vi "Engine Out - Direct Injectors.vi"(7 "Rail Pressure [bar]":sgl, 10 "DI Timings (DBTDC)":T3[](array[typedef]), 11 "DI Quantities (mg/inj)":T2[](array[typedef])) -> (0 "Injector 5":T1, 1 "Injector 6":T1, 2 "Injector 7":T1, 3 "Injector 8":T1, 4 "Injector 4":T1, 6 "Injector 3":T1, 8 "Injector 2":T1, 9 "Injector 1":T1)   [LabVIEW 2015, in "ECS-RT.lvlib"]
uses:
  ECS-RT.lvlib
  Typedefs/Control Outputs/Injection Timing.ctl
  Typedefs/Control Outputs/Injection Quantity.ctl
  Typedefs/Raw Outputs/DI.ctl
  ECS-Shared.lvlib
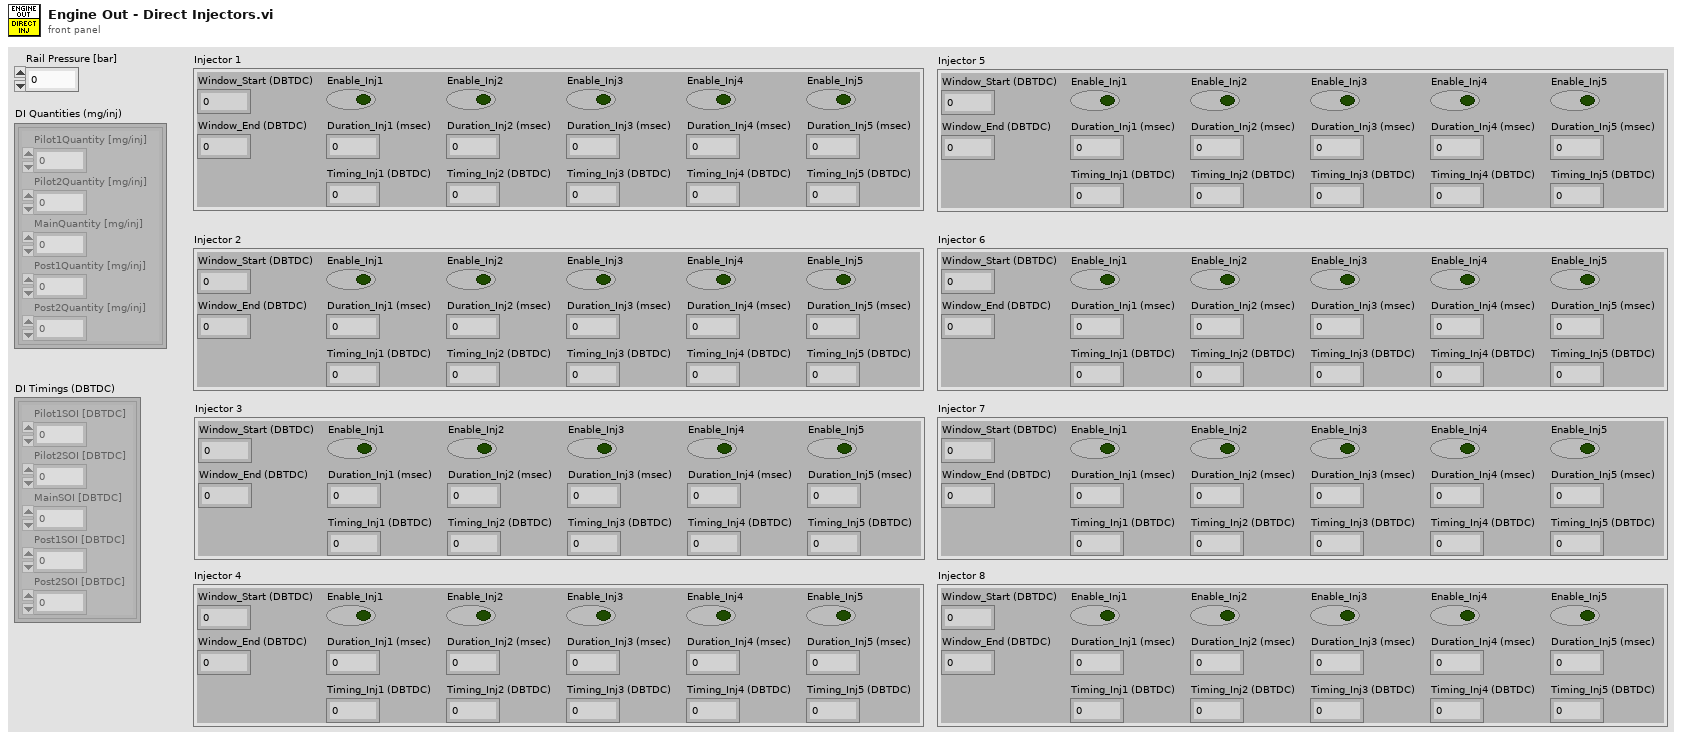
[diagram p1: front panel]
types:
  T1 = typedef "ECS-Shared.lvlib/DI.ctl" = cluster{"Window_Start (DBTDC)":sgl, "Window_End (DBTDC)":sgl, "Enable_Inj1":bool, "Duration_Inj1 (msec)":sgl, "Timing_Inj1 (DBTDC)":sgl, "Enable_Inj2":bool, "Duration_Inj2 (msec)":sgl, "Timing_Inj2 (DBTDC)":sgl, "Enable_Inj3":bool, "Duration_Inj3 (msec)":sgl, "Timing_Inj3 (DBTDC)":sgl, "Enable_Inj4":bool, "Duration_Inj4 (msec)":sgl, "Timing_Inj4 (DBTDC)":sgl, "Enable_Inj5":bool, "Duration_Inj5 (msec)":sgl, "Timing_Inj5 (DBTDC)":sgl}
  T2 = typedef "ECS-Shared.lvlib/Injection Quantity.ctl" = cluster{"Pilot1Quantity [mg/inj]":sgl, "Pilot2Quantity [mg/inj]":sgl, "MainQuantity [mg/inj]":sgl, "Post1Quantity [mg/inj]":sgl, "Post2Quantity [mg/inj]":sgl}
  T3 = typedef "ECS-Shared.lvlib/Injection Timing.ctl" = cluster{"Pilot1SOI [DBTDC]":sgl, "Pilot2SOI [DBTDC]":sgl, "MainSOI [DBTDC]":sgl, "Post1SOI [DBTDC]":sgl, "Post2SOI [DBTDC]":sgl}
  T4 = cluster{"Pilot1Duration [msec]":sgl, "Pilot2Duration [msec]":sgl, "MainDuration [msec]":sgl, "Post1Duration [msec]":sgl, "Post2Duration [msec]":sgl}
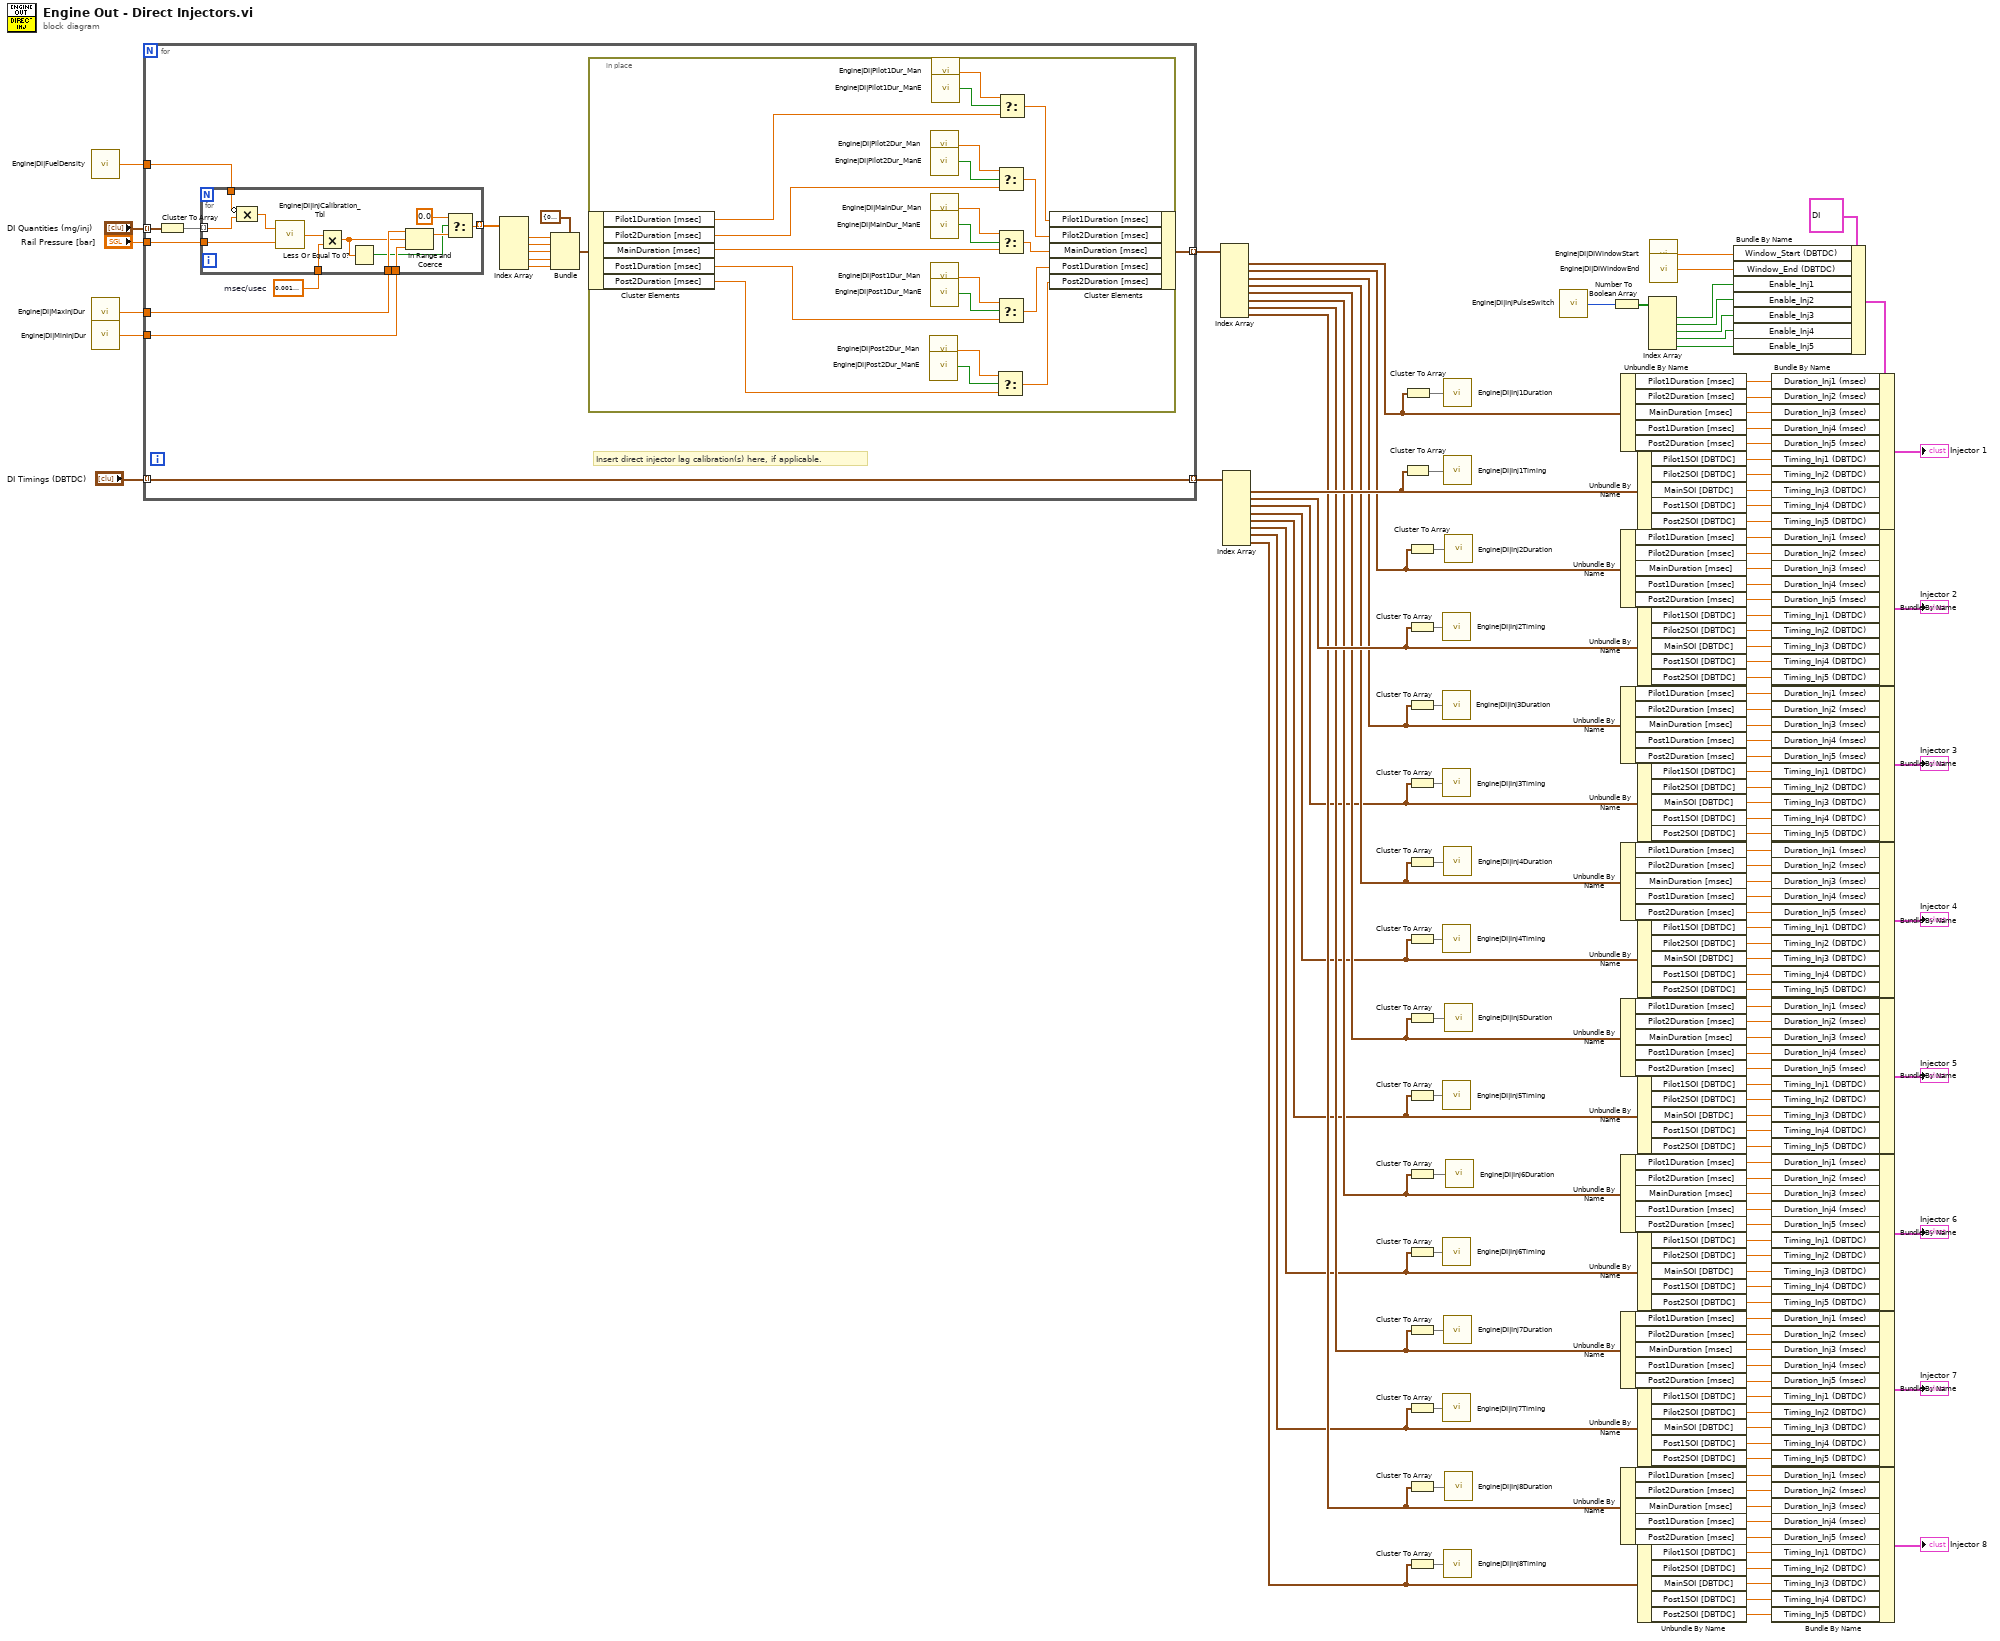
[diagram p0: block diagram]
diagram:
  n1 = call "Engine|DI|FuelDensity"() -> ("Value"=w3:sgl)
  n2 = call "Engine|DI|MaxInjDur"() -> ("Value"=w2:sgl)
  n3 = call "Engine|DI|MinInjDur"() -> ("Value"=w1:sgl)
  n4 = for {
    tunnel: "DI Quantities (mg/inj)" -> [w147] mode=indexing
    tunnel: [w145] -> w37 mode=indexing
    tunnel: "Rail Pressure [bar]" -> [w144]
    tunnel: "DI Timings (DBTDC)" -> [w143] mode=indexing
    tunnel: [w143] -> w38 mode=indexing
    tunnel: w3 -> [w142]
    tunnel: w2 -> [w141]
    tunnel: w1 -> [w140]
    w149 = sgl 0.001  # msec/usec
    # "Insert direct injector lag calibration(s) here, if applicable."
    n5 = Cluster To Array(cluster=w147) -> (array=w148:sgl[])
    n6 = for {
      tunnel: [w180] -> w150 mode=indexing
      tunnel: w149 -> [w188]
      tunnel: w148 -> [w185] mode=indexing
      tunnel: w144 -> [w187]
      tunnel: w142 -> [w186]
      tunnel: w141 -> [w183]
      tunnel: w140 -> [w182]
      n7 = Compound Arithmetic op=MULTIPLY(invert w186, w185) -> (w184:sgl)
      n8 = call "Engine|DI|InjCalibration_Tbl"("Y Index"=w187, "X Index"=w184) -> ("Z"=w189:sgl)
      n9 = Multiply(x=w189, y=w188) -> (x*y=w181:sgl)
      n10 = Less Or Equal To 0?(x=w181) -> (x <= 0?=w177:bool)
      n11 = In Range and Coerce(upper limit=w183, x=w181, lower limit=w182) -> (coerced(x)=w179:sgl)  [unwired: 1 out]
      n12 = Select(t=sgl 0.0, s=w177, f=w179) -> (s? t:f=w180:sgl)
    }
    n13 = Index Array(array=w150) -> (element #1=w151:sgl, element #2=w152:sgl, element #3=w153:sgl, element #4=w154:sgl, element #5=w155:sgl)  [unwired: 5 in]
    n14 = Bundle(cluster=T4 {"Pilot1Duration [msec]"=0.0, "Pilot2Duration [msec]"=0.0, "MainDuration [msec]"=0.0, "Post1Duration [msec]"=0.0, "Post2Duration [msec]"=0.0} ("DI Injection Durations (msec)"), "Pilot1Duration [msec]"=w151, "Pilot2Duration [msec]"=w152, "MainDuration [msec]"=w153, "Post1Duration [msec]"=w154, "Post2Duration [msec]"=w155) -> (w146:T4)
    n15 = in-place {
      n16 = in-place-cluster #1(w146) -> ("Pilot1Duration [msec]"=w166:sgl, "Pilot2Duration [msec]"=w165:sgl, "MainDuration [msec]"=w164:sgl, "Post1Duration [msec]"=w163:sgl, "Post2Duration [msec]"=w162:sgl)
      n17 = call "Engine|DI|Post2Dur_Man"() -> ("Value"=w175:sgl)
      n18 = call "Engine|DI|Post2Dur_ManE"() -> ("Value"=w176:bool)
      n19 = call "Engine|DI|Pilot2Dur_Man"() -> ("Value"=w171:sgl)
      n20 = call "Engine|DI|Pilot2Dur_ManE"() -> ("Value"=w172:bool)
      n21 = call "Engine|DI|MainDur_Man"() -> ("Value"=w167:sgl)
      n22 = call "Engine|DI|MainDur_ManE"() -> ("Value"=w168:bool)
      n23 = call "Engine|DI|Post1Dur_Man"() -> ("Value"=w173:sgl)
      n24 = call "Engine|DI|Post1Dur_ManE"() -> ("Value"=w174:bool)
      n25 = call "Engine|DI|Pilot1Dur_Man"() -> ("Value"=w169:sgl)
      n26 = call "Engine|DI|Pilot1Dur_ManE"() -> ("Value"=w170:bool)
      n27 = Select(t=w175, s=w176, f=w162) -> (s? t:f=w157:sgl)
      n28 = Select(t=w171, s=w172, f=w165) -> (s? t:f=w160:sgl)
      n29 = Select(t=w167, s=w168, f=w164) -> (s? t:f=w159:sgl)
      n30 = Select(t=w173, s=w174, f=w163) -> (s? t:f=w158:sgl)
      n31 = Select(t=w169, s=w170, f=w166) -> (s? t:f=w161:sgl)
      n32 = in-place-cluster #1("Pilot1Duration [msec]"=w161, "Pilot2Duration [msec]"=w160, "MainDuration [msec]"=w159, "Post1Duration [msec]"=w158, "Post2Duration [msec]"=w157) -> (w145:T4)
    }
  }
  n33 = Index Array(array=w37) -> (element #1=w19:T4, element #2=w17:T4, element #3=w4:T4, element #4=w6:T4, element #5=w8:T4, element #6=w10:T4, element #7=w12:T4, element #8=w14:T4)  [unwired: 8 in]
  n34 = Index Array(array=w38) -> (element #1=w18:T3, element #2=w16:T3, element #3=w5:T3, element #4=w7:T3, element #5=w9:T3, element #6=w11:T3, element #7=w13:T3, element #8=w15:T3)  [unwired: 8 in]
  n35 = Cluster To Array(cluster=w18) -> (array=w27:sgl[])
  n36 = Cluster To Array(cluster=w19) -> (array=w29:sgl[])
  n37 = Cluster To Array(cluster=w17) -> (array=w30:sgl[])
  n38 = Cluster To Array(cluster=w16) -> (array=w20:sgl[])
  n39 = Cluster To Array(cluster=w4) -> (array=w28:sgl[])
  n40 = Cluster To Array(cluster=w5) -> (array=w21:sgl[])
  n41 = Cluster To Array(cluster=w6) -> (array=w31:sgl[])
  n42 = Cluster To Array(cluster=w7) -> (array=w22:sgl[])
  n43 = Cluster To Array(cluster=w8) -> (array=w32:sgl[])
  n44 = Cluster To Array(cluster=w9) -> (array=w23:sgl[])
  n45 = Cluster To Array(cluster=w10) -> (array=w33:sgl[])
  n46 = Cluster To Array(cluster=w11) -> (array=w24:sgl[])
  n47 = Cluster To Array(cluster=w12) -> (array=w34:sgl[])
  n48 = Cluster To Array(cluster=w13) -> (array=w25:sgl[])
  n49 = Cluster To Array(cluster=w14) -> (array=w35:sgl[])
  n50 = Cluster To Array(cluster=w15) -> (array=w26:sgl[])
  n51 = call "Engine|DI|Inj2Timing"("Value"=w20) -> ()
  n52 = call "Engine|DI|Inj3Duration"("Value"=w28) -> ()
  n53 = call "Engine|DI|Inj3Timing"("Value"=w21) -> ()
  n54 = call "Engine|DI|Inj4Timing"("Value"=w22) -> ()
  n55 = call "Engine|DI|Inj5Timing"("Value"=w23) -> ()
  n56 = call "Engine|DI|Inj6Timing"("Value"=w24) -> ()
  n57 = call "Engine|DI|Inj7Timing"("Value"=w25) -> ()
  n58 = call "Engine|DI|Inj1Duration"("Value"=w29) -> ()
  n59 = call "Engine|DI|Inj1Timing"("Value"=w27) -> ()
  n60 = call "Engine|DI|Inj4Duration"("Value"=w31) -> ()
  n61 = call "Engine|DI|Inj7Duration"("Value"=w34) -> ()
  n62 = call "Engine|DI|Inj8Timing"("Value"=w26) -> ()
  n63 = call "Engine|DI|Inj2Duration"("Value"=w30) -> ()
  n64 = call "Engine|DI|Inj5Duration"("Value"=w32) -> ()
  n65 = call "Engine|DI|Inj8Duration"("Value"=w35) -> ()
  n66 = call "Engine|DI|Inj6Duration"("Value"=w33) -> ()
  n67 = call "Engine|DI|InjPulseSwitch"() -> ("Value"=w131:u8)
  n68 = Number To Boolean Array(number=w131) -> (Boolean array=w132:bool[])
  n69 = Unbundle By Name(w19) -> ("Pilot1Duration [msec]"=w79:sgl, "Pilot2Duration [msec]"=w80:sgl, "MainDuration [msec]"=w81:sgl, "Post1Duration [msec]"=w82:sgl, "Post2Duration [msec]"=w83:sgl)
  n70 = Unbundle By Name(w17) -> ("Pilot1Duration [msec]"=w84:sgl, "Pilot2Duration [msec]"=w88:sgl, "MainDuration [msec]"=w87:sgl, "Post1Duration [msec]"=w86:sgl, "Post2Duration [msec]"=w85:sgl)
  n71 = Unbundle By Name(w4) -> ("Pilot1Duration [msec]"=w89:sgl, "Pilot2Duration [msec]"=w90:sgl, "MainDuration [msec]"=w91:sgl, "Post1Duration [msec]"=w92:sgl, "Post2Duration [msec]"=w93:sgl)
  n72 = Unbundle By Name(w6) -> ("Pilot1Duration [msec]"=w94:sgl, "Pilot2Duration [msec]"=w95:sgl, "MainDuration [msec]"=w96:sgl, "Post1Duration [msec]"=w97:sgl, "Post2Duration [msec]"=w98:sgl)
  n73 = Unbundle By Name(w8) -> ("Pilot1Duration [msec]"=w99:sgl, "Pilot2Duration [msec]"=w100:sgl, "MainDuration [msec]"=w101:sgl, "Post1Duration [msec]"=w102:sgl, "Post2Duration [msec]"=w103:sgl)
  n74 = Unbundle By Name(w10) -> ("Pilot1Duration [msec]"=w104:sgl, "Pilot2Duration [msec]"=w105:sgl, "MainDuration [msec]"=w106:sgl, "Post1Duration [msec]"=w107:sgl, "Post2Duration [msec]"=w108:sgl)
  n75 = Unbundle By Name(w12) -> ("Pilot1Duration [msec]"=w109:sgl, "Pilot2Duration [msec]"=w110:sgl, "MainDuration [msec]"=w111:sgl, "Post1Duration [msec]"=w112:sgl, "Post2Duration [msec]"=w113:sgl)
  n76 = Unbundle By Name(w14) -> ("Pilot1Duration [msec]"=w114:sgl, "Pilot2Duration [msec]"=w115:sgl, "MainDuration [msec]"=w116:sgl, "Post1Duration [msec]"=w117:sgl, "Post2Duration [msec]"=w118:sgl)
  n77 = Unbundle By Name(w18) -> ("Pilot1SOI [DBTDC]"=w78:sgl, "Pilot2SOI [DBTDC]"=w77:sgl, "MainSOI [DBTDC]"=w76:sgl, "Post1SOI [DBTDC]"=w75:sgl, "Post2SOI [DBTDC]"=w74:sgl)
  n78 = Unbundle By Name(w16) -> ("Pilot1SOI [DBTDC]"=w69:sgl, "Pilot2SOI [DBTDC]"=w70:sgl, "MainSOI [DBTDC]"=w71:sgl, "Post1SOI [DBTDC]"=w72:sgl, "Post2SOI [DBTDC]"=w73:sgl)
  n79 = Unbundle By Name(w5) -> ("Pilot1SOI [DBTDC]"=w68:sgl, "Pilot2SOI [DBTDC]"=w67:sgl, "MainSOI [DBTDC]"=w66:sgl, "Post1SOI [DBTDC]"=w65:sgl, "Post2SOI [DBTDC]"=w64:sgl)
  n80 = Unbundle By Name(w7) -> ("Pilot1SOI [DBTDC]"=w59:sgl, "Pilot2SOI [DBTDC]"=w60:sgl, "MainSOI [DBTDC]"=w61:sgl, "Post1SOI [DBTDC]"=w62:sgl, "Post2SOI [DBTDC]"=w63:sgl)
  n81 = Unbundle By Name(w9) -> ("Pilot1SOI [DBTDC]"=w39:sgl, "Pilot2SOI [DBTDC]"=w40:sgl, "MainSOI [DBTDC]"=w41:sgl, "Post1SOI [DBTDC]"=w42:sgl, "Post2SOI [DBTDC]"=w43:sgl)
  n82 = Unbundle By Name(w11) -> ("Pilot1SOI [DBTDC]"=w48:sgl, "Pilot2SOI [DBTDC]"=w47:sgl, "MainSOI [DBTDC]"=w46:sgl, "Post1SOI [DBTDC]"=w45:sgl, "Post2SOI [DBTDC]"=w44:sgl)
  n83 = Unbundle By Name(w13) -> ("Pilot1SOI [DBTDC]"=w49:sgl, "Pilot2SOI [DBTDC]"=w50:sgl, "MainSOI [DBTDC]"=w51:sgl, "Post1SOI [DBTDC]"=w52:sgl, "Post2SOI [DBTDC]"=w53:sgl)
  n84 = Unbundle By Name(w15) -> ("Pilot1SOI [DBTDC]"=w58:sgl, "Pilot2SOI [DBTDC]"=w57:sgl, "MainSOI [DBTDC]"=w56:sgl, "Post1SOI [DBTDC]"=w55:sgl, "Post2SOI [DBTDC]"=w54:sgl)
  n85 = Index Array(array=w132) -> (element #1=w134:bool, element #2=w137:bool, element #3=w136:bool, element #4=w135:bool, element #5=w133:bool)  [unwired: 5 in]
  n86 = call "Engine|DI|DIWindowStart"() -> ("Value"=w139:sgl)
  n87 = call "Engine|DI|DIWindowEnd"() -> ("Value"=w138:sgl)
  n88 = Bundle By Name(cluster=T1 {"Window_Start (DBTDC)"=0.0, "Window_End (DBTDC)"=0.0, "Enable_Inj1"=FALSE, "Duration_Inj1 (msec)"=0.0, "Timing_Inj1 (DBTDC)"=0.0, "Enable_Inj2"=FALSE, "Duration_Inj2 (msec)"=0.0, "Timing_Inj2 (DBTDC)"=0.0, "Enable_Inj3"=FALSE, "Duration_Inj3 (msec)"=0.0, "Timing_Inj3 (DBTDC)"=0.0, "Enable_Inj4"=FALSE, "Duration_Inj4 (msec)"=0.0, "Timing_Inj4 (DBTDC)"=0.0, "Enable_Inj5"=FALSE, "Duration_Inj5 (msec)"=0.0, "Timing_Inj5 (DBTDC)"=0.0} ("DI"), "Window_Start (DBTDC)"=w139, "Window_End (DBTDC)"=w138, "Enable_Inj1"=w134, "Enable_Inj2"=w137, "Enable_Inj3"=w136, "Enable_Inj4"=w135, "Enable_Inj5"=w133) -> (w36:T1)
  n89 = Bundle By Name(cluster=w36, "Duration_Inj1 (msec)"=w79, "Duration_Inj2 (msec)"=w80, "Duration_Inj3 (msec)"=w81, "Duration_Inj4 (msec)"=w82, "Duration_Inj5 (msec)"=w83, "Timing_Inj1 (DBTDC)"=w78, "Timing_Inj2 (DBTDC)"=w77, "Timing_Inj3 (DBTDC)"=w76, "Timing_Inj4 (DBTDC)"=w75, "Timing_Inj5 (DBTDC)"=w74) -> (→"Injector 1":T1)
  n90 = Bundle By Name(cluster=w36, "Duration_Inj1 (msec)"=w84, "Duration_Inj2 (msec)"=w88, "Duration_Inj3 (msec)"=w87, "Duration_Inj4 (msec)"=w86, "Duration_Inj5 (msec)"=w85, "Timing_Inj1 (DBTDC)"=w69, "Timing_Inj2 (DBTDC)"=w70, "Timing_Inj3 (DBTDC)"=w71, "Timing_Inj4 (DBTDC)"=w72, "Timing_Inj5 (DBTDC)"=w73) -> (→"Injector 2":T1)
  n91 = Bundle By Name(cluster=w36, "Duration_Inj1 (msec)"=w89, "Duration_Inj2 (msec)"=w90, "Duration_Inj3 (msec)"=w91, "Duration_Inj4 (msec)"=w92, "Duration_Inj5 (msec)"=w93, "Timing_Inj1 (DBTDC)"=w68, "Timing_Inj2 (DBTDC)"=w67, "Timing_Inj3 (DBTDC)"=w66, "Timing_Inj4 (DBTDC)"=w65, "Timing_Inj5 (DBTDC)"=w64) -> (→"Injector 3":T1)
  n92 = Bundle By Name(cluster=w36, "Duration_Inj1 (msec)"=w94, "Duration_Inj2 (msec)"=w95, "Duration_Inj3 (msec)"=w96, "Duration_Inj4 (msec)"=w97, "Duration_Inj5 (msec)"=w98, "Timing_Inj1 (DBTDC)"=w59, "Timing_Inj2 (DBTDC)"=w60, "Timing_Inj3 (DBTDC)"=w61, "Timing_Inj4 (DBTDC)"=w62, "Timing_Inj5 (DBTDC)"=w63) -> (→"Injector 4":T1)
  n93 = Bundle By Name(cluster=w36, "Duration_Inj1 (msec)"=w99, "Duration_Inj2 (msec)"=w100, "Duration_Inj3 (msec)"=w101, "Duration_Inj4 (msec)"=w102, "Duration_Inj5 (msec)"=w103, "Timing_Inj1 (DBTDC)"=w39, "Timing_Inj2 (DBTDC)"=w40, "Timing_Inj3 (DBTDC)"=w41, "Timing_Inj4 (DBTDC)"=w42, "Timing_Inj5 (DBTDC)"=w43) -> (→"Injector 5":T1)
  n94 = Bundle By Name(cluster=w36, "Duration_Inj1 (msec)"=w104, "Duration_Inj2 (msec)"=w105, "Duration_Inj3 (msec)"=w106, "Duration_Inj4 (msec)"=w107, "Duration_Inj5 (msec)"=w108, "Timing_Inj1 (DBTDC)"=w48, "Timing_Inj2 (DBTDC)"=w47, "Timing_Inj3 (DBTDC)"=w46, "Timing_Inj4 (DBTDC)"=w45, "Timing_Inj5 (DBTDC)"=w44) -> (→"Injector 6":T1)
  n95 = Bundle By Name(cluster=w36, "Duration_Inj1 (msec)"=w109, "Duration_Inj2 (msec)"=w110, "Duration_Inj3 (msec)"=w111, "Duration_Inj4 (msec)"=w112, "Duration_Inj5 (msec)"=w113, "Timing_Inj1 (DBTDC)"=w49, "Timing_Inj2 (DBTDC)"=w50, "Timing_Inj3 (DBTDC)"=w51, "Timing_Inj4 (DBTDC)"=w52, "Timing_Inj5 (DBTDC)"=w53) -> (→"Injector 7":T1)
  n96 = Bundle By Name(cluster=w36, "Duration_Inj1 (msec)"=w114, "Duration_Inj2 (msec)"=w115, "Duration_Inj3 (msec)"=w116, "Duration_Inj4 (msec)"=w117, "Duration_Inj5 (msec)"=w118, "Timing_Inj1 (DBTDC)"=w58, "Timing_Inj2 (DBTDC)"=w57, "Timing_Inj3 (DBTDC)"=w56, "Timing_Inj4 (DBTDC)"=w55, "Timing_Inj5 (DBTDC)"=w54) -> (→"Injector 8":T1)
